vi "Position Country Enum.vi"(8 "error in (no error)":errorcluster, 10 "Previous String":refnum<vi>, 11 "Country Enum":refnum<vi>) -> (0 "error out":errorcluster)   [LabVIEW 2014]
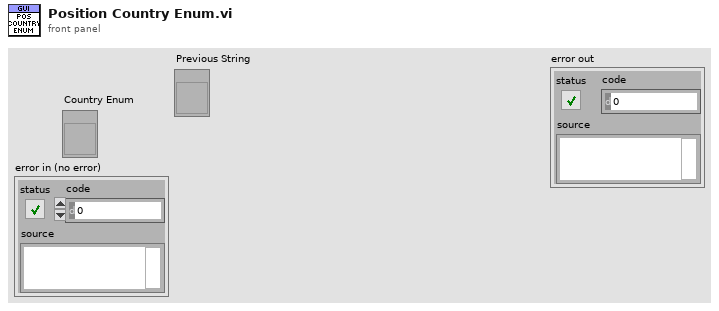
[diagram p1: front panel]
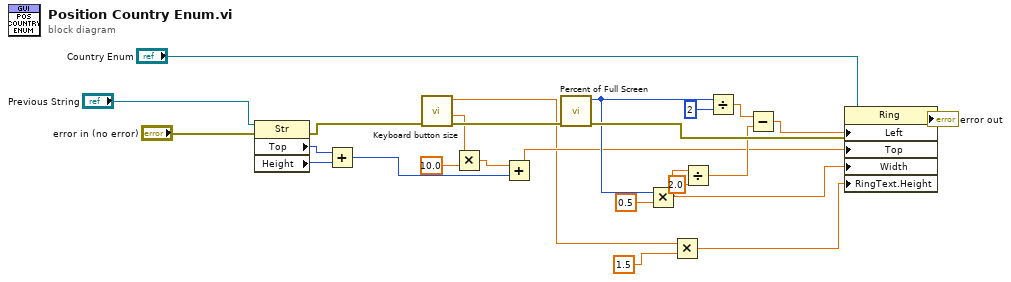
[diagram p0: block diagram]
diagram:
  n1 = property class="Str"(reference="Previous String", error in="error in (no error)") -> (error out=w10:errorcluster, "Top"=w12:i32, "Height"=w11:u32)  [unwired: 1 out]
  n2 = Add(x=w12, y=w11) -> (x+y=w8:u32)
  n3 = call "Keyboard button size.vi"("error in (no error)"=w10) -> ("error out"=w9:errorcluster, "Key Spacing"=w5:dbl, "Key Height"=w3:dbl)  [unwired: 7 in, 1 out]
  n4 = Multiply(x=w5, y=10.0) -> (x*y=w6:dbl)
  n5 = Add(x=w6, y=w8) -> (x+y=w7:dbl)
  n6 = call "Percent of Full Screen.vi"("error in (no error)"=w9) -> ("error out"=w23:errorcluster, "Right"=w20:i16)  [unwired: 8 in, 1 out]
  n7 = Multiply(x=w20, y=0.5) -> (x*y=w17:dbl)
  n8 = Multiply(x=w3, y=1.5) -> (x*y=w1:dbl)
  n9 = Divide(x=w17, y=2.0) -> (x/y=w15:dbl)
  n10 = Divide(x=w20, y=i16 2) -> (x/y=w24:dbl)
  n11 = Subtract(x=w24, y=w15) -> (x-y=w22:dbl)
  n12 = property class="Ring"(reference="Country Enum", error in=w23, "Left"=w22, "Top"=w7, "Width"=w17, "RingText.Height"=w1) -> (error out=→"error out":errorcluster)  [unwired: 1 out]
